vi "Emergency_Safe_Shutdown_JT.vi"(8 "error in":errorcluster, 11 "connection ID":refnum<k5>) -> (0 "error out":errorcluster)   [LabVIEW 2016]
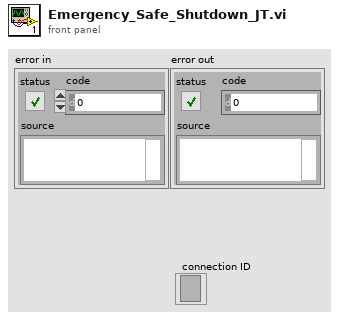
[diagram p1: front panel]
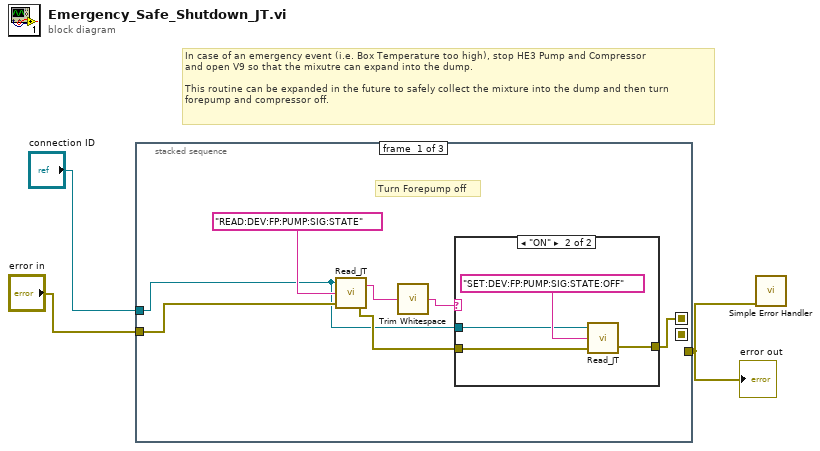
[diagram p0: block diagram]
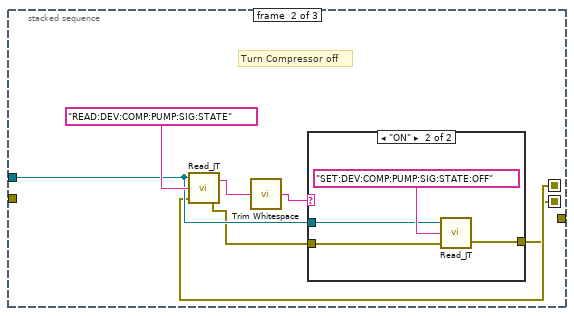
[diagram p3: hidden frame]
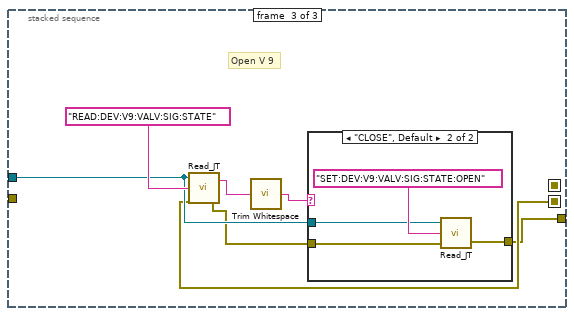
[diagram p5: hidden frame]
diagram:
  # "In case of an emergency event (i.e. Box Temperature too high), stop HE3 Pump and Compressor\nand open V9 so that the mixutre can expand into the dump.\n\nThis routine can be expanded in the future to safely collect the mixture into the dump and then turn \nforepump and compressor off."
  n1 = stacked-sequence {
    seq-local: [_ w16 _] -> [_ _ w29]
    seq-local: [w4 _ _] -> [_ w17 _]
    tunnel: "connection ID" -> [w5 w21 w33]
    tunnel: "error in" -> [w6 _ _]
    tunnel: [_ _ w28] -> w1
    frame #0 {
      # "Turn Forepump off"
      n2 = call "Read_JT.vi"("error in"=w6, "Write"="READ:DEV:FP:PUMP:SIG:STATE", "connection ID"=w5) -> ("error out"=w9:errorcluster, "Read"=w8:string)
      n3 = call <vilib>:"Trim Whitespace.vi"("string"=w8) -> ("trimmed string"=w7:string)  [unwired: 1 in]
      n4 = case shown="\"ON\"" w7 {
        tunnel: w5 -> [_ w14]
        tunnel: w9 -> [w11 w13]
        tunnel: [w11 w12] -> w4
        frame "OFF", Default {
        }
        frame "ON" {
          n5 = call "Read_JT.vi"("error in"=w13, "Write"="SET:DEV:FP:PUMP:SIG:STATE:OFF", "connection ID"=w14) -> ("error out"=w12:errorcluster)  [unwired: 1 out]
        }
      }
    }
    frame #1 {
      # "Turn Compressor off"
      n6 = call "Read_JT.vi"("error in"=w17, "Write"="READ:DEV:COMP:PUMP:SIG:STATE", "connection ID"=w21) -> ("error out"=w20:errorcluster, "Read"=w19:string)
      n7 = call <vilib>:"Trim Whitespace.vi"("string"=w19) -> ("trimmed string"=w18:string)  [unwired: 1 in]
      n8 = case shown="\"ON\"" w18 {
        tunnel: w21 -> [_ w26]
        tunnel: w20 -> [w23 w25]
        tunnel: [w23 w24] -> w16
        frame "OFF", Default {
        }
        frame "ON" {
          n9 = call "Read_JT.vi"("error in"=w25, "Write"="SET:DEV:COMP:PUMP:SIG:STATE:OFF", "connection ID"=w26) -> ("error out"=w24:errorcluster)  [unwired: 1 out]
        }
      }
    }
    frame #2 {
      # "Open V 9"
      n10 = call "Read_JT.vi"("error in"=w29, "Write"="READ:DEV:V9:VALV:SIG:STATE", "connection ID"=w33) -> ("error out"=w32:errorcluster, "Read"=w31:string)
      n11 = call <vilib>:"Trim Whitespace.vi"("string"=w31) -> ("trimmed string"=w30:string)  [unwired: 1 in]
      n12 = case shown="\"CLOSE\", Default" w30 {
        tunnel: w33 -> [_ w38]
        tunnel: w32 -> [w35 w37]
        tunnel: [w35 w36] -> w28
        frame "OPEN" {
        }
        frame "CLOSE", Default {
          n13 = call "Read_JT.vi"("error in"=w37, "Write"="SET:DEV:V9:VALV:SIG:STATE:OPEN", "connection ID"=w38) -> ("error out"=w36:errorcluster)  [unwired: 1 out]
        }
      }
    }
  }
  "error out" <- w1
  n14 = call <vilib>:"Simple Error Handler.vi"("error in (no error)"=w1) -> ()  [unwired: 4 in, 5 out]
